vi "Wings_AntiBack.vi"(3 "Toggle":bool, 4 "Update?":bool, 5 "MtrPwrIn":dbl) -> (0 "State":bool, 2 "MtrPwrOut":dbl)   [LabVIEW 2017]
uses:
  <vilib>/Rock Robotics/WPI/Solenoid/Deprecated/WPI_SolenoidSetBool.vi
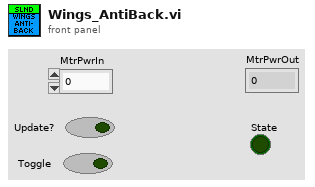
[diagram p1: front panel]
types:
  T1 = typedef "WPI_SolenoidDevRef.ctl" = cluster{"DevStatus":errorcluster, "Pneumatics Control Module":u8, "Forward Solenoid Channel":T2, "Reverse Solenoid Channel":T2}
  T2 = typedef "WPI_SolenoidChannel.ctl" = enum8{"Solenoid 0", "Solenoid 1", "Solenoid 2", "Solenoid 3", "Solenoid 4", "Solenoid 5", "Solenoid 6", "Solenoid 7", "Invalid"}
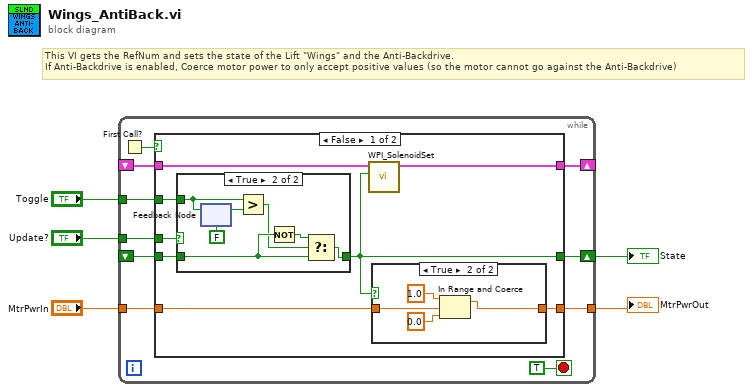
[diagram p0: block diagram]
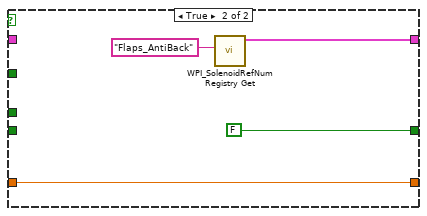
[diagram p4: hidden frame]
diagram:
  # "This VI gets the RefNum and sets the state of the Lift \"Wings\" and the Anti-Backdrive.\nIf Anti-Backdrive is enabled, Coerce motor power to only accept positive values (so the motor cannot go against the Anti-Backdrive)"
  n1 = while {
    shift-right: [w12] -> w2
    shift-left: _ -> [w13]
    shift-right: [w11] -> _
    shift-left: _ -> [w10]
    tunnel: "Toggle" -> [w9]
    tunnel: "MtrPwrIn" -> [w8]
    tunnel: [w7] -> w3
    tunnel: "Update?" -> [w6]
    stop <- TRUE stop-if-true
    n2 = First Call?() -> (First Call?: T/F=w14:bool)
    n3 = case shown="False" w14 {
      tunnel: w13 -> [w21 _]
      tunnel: [w18 FALSE ("Shift")] -> w12
      tunnel: [w22 w39] -> w11
      tunnel: w10 -> [w23 _]
      tunnel: w9 -> [w16 _]
      tunnel: w8 -> [w20 w37]
      tunnel: [w19 w37] -> w7
      tunnel: w6 -> [w17 _]
      frame False {
        n4 = case shown="True" w17 {
          tunnel: w21 -> [w24 w30]
          tunnel: [w24 w26] -> w18
          tunnel: w16 -> [_ w25]
          frame False {
          }
          frame True {
            n5 = feedback #1(FALSE) -> (w29:bool)
            n6 = feedback-in #1(w25) -> ()
            n7 = Greater?(x=w25, y=w29) -> (0:w27:bool)
            n8 = Not(x=w30) -> (.not. x?=w31:bool)
            n9 = Select(t=w31, s=w27, f=w30) -> (s? t:f=w26:bool)
          }
        }
        n10 = call-poly <vilib>:"WPI_SolenoidSet.vi"("Value"=w18, "SolenoidDevRef"=w23) -> ("SolenoidDevRef"=w22:T1)  [unwired: 8 in, 1 out]
        n11 = case shown="True" w18 {
          tunnel: w20 -> [w32 w34]
          tunnel: [w32 w33] -> w19
          frame False {
          }
          frame True {
            n12 = In Range and Coerce(upper limit=1.0, x=w34, lower limit=0.0) -> (coerced(x)=w33:dbl)  [unwired: 1 out]
          }
        }
      }
      frame True {
        n13 = call <vilib>:"WPI_SolenoidRefNum Registry Get.vi"("refnum name"="Flaps_AntiBack") -> ("SolenoidDevRef"=w39:T1)  [unwired: 9 in, 1 out]
      }
    }
  }
  "MtrPwrOut" <- w3
  "State" <- w2
